vi "ReadPropertiesAccessor.vi"(8 "error in (no error)":errorcluster, 11 "VXMx2 in":refnum<class "VXMx2.lvclass">) -> (0 "error out":errorcluster, 1 "Homed=T":bool, 3 "VXMx2 out":refnum<class "VXMx2.lvclass">)   [LabVIEW 2019, in "VXMx2.lvclass"]
uses:
  VXMx2.lvclass
  VXMx2.lvclass/VXMx2.ctl
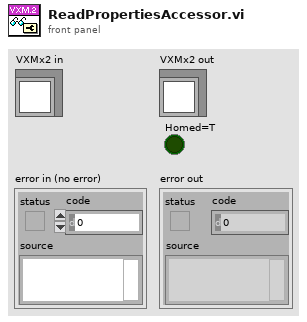
[diagram p1: front panel]
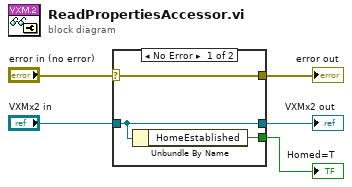
[diagram p0: block diagram]
diagram:
  n1 = case shown="No Error" "error in (no error)" {
    selector: "error in (no error)" -> [w8 w10]
    tunnel: [w8 w10] -> w4
    tunnel: [w7 w9] -> w2
    tunnel: "VXMx2 in" -> [w7 w9]
    tunnel: [w6 _] -> w1
    frame No Error {
      n2 = Unbundle By Name(w7) -> ("HomeEstablished"=w6:bool)
    }
    frame Error {
    }
  }
  "error out" <- w4
  "VXMx2 out" <- w2
  "Homed=T" <- w1
